vi "GetExecutableConfigurationFilePath.vi"(8 "Error In":errorcluster, 10 "Application Name":string, 11 "VI Path":path) -> (0 "Error Out":errorcluster, 3 "Executable Config File Path":path)   [LabVIEW 2012, in "LV-Utilities.lvlib"]
uses:
  LV-Utilities.lvlib
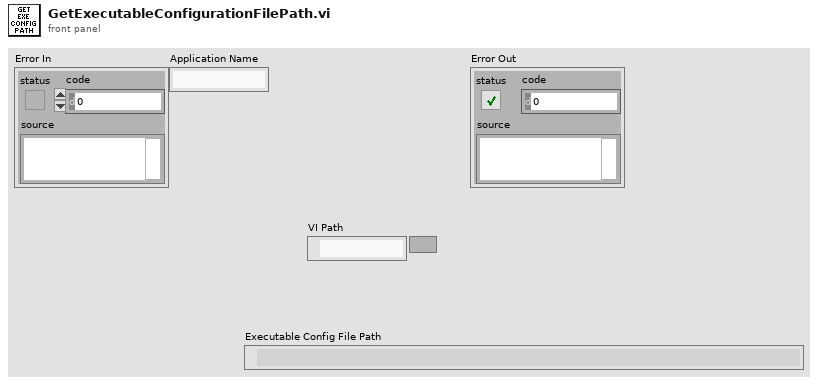
[diagram p1: front panel]
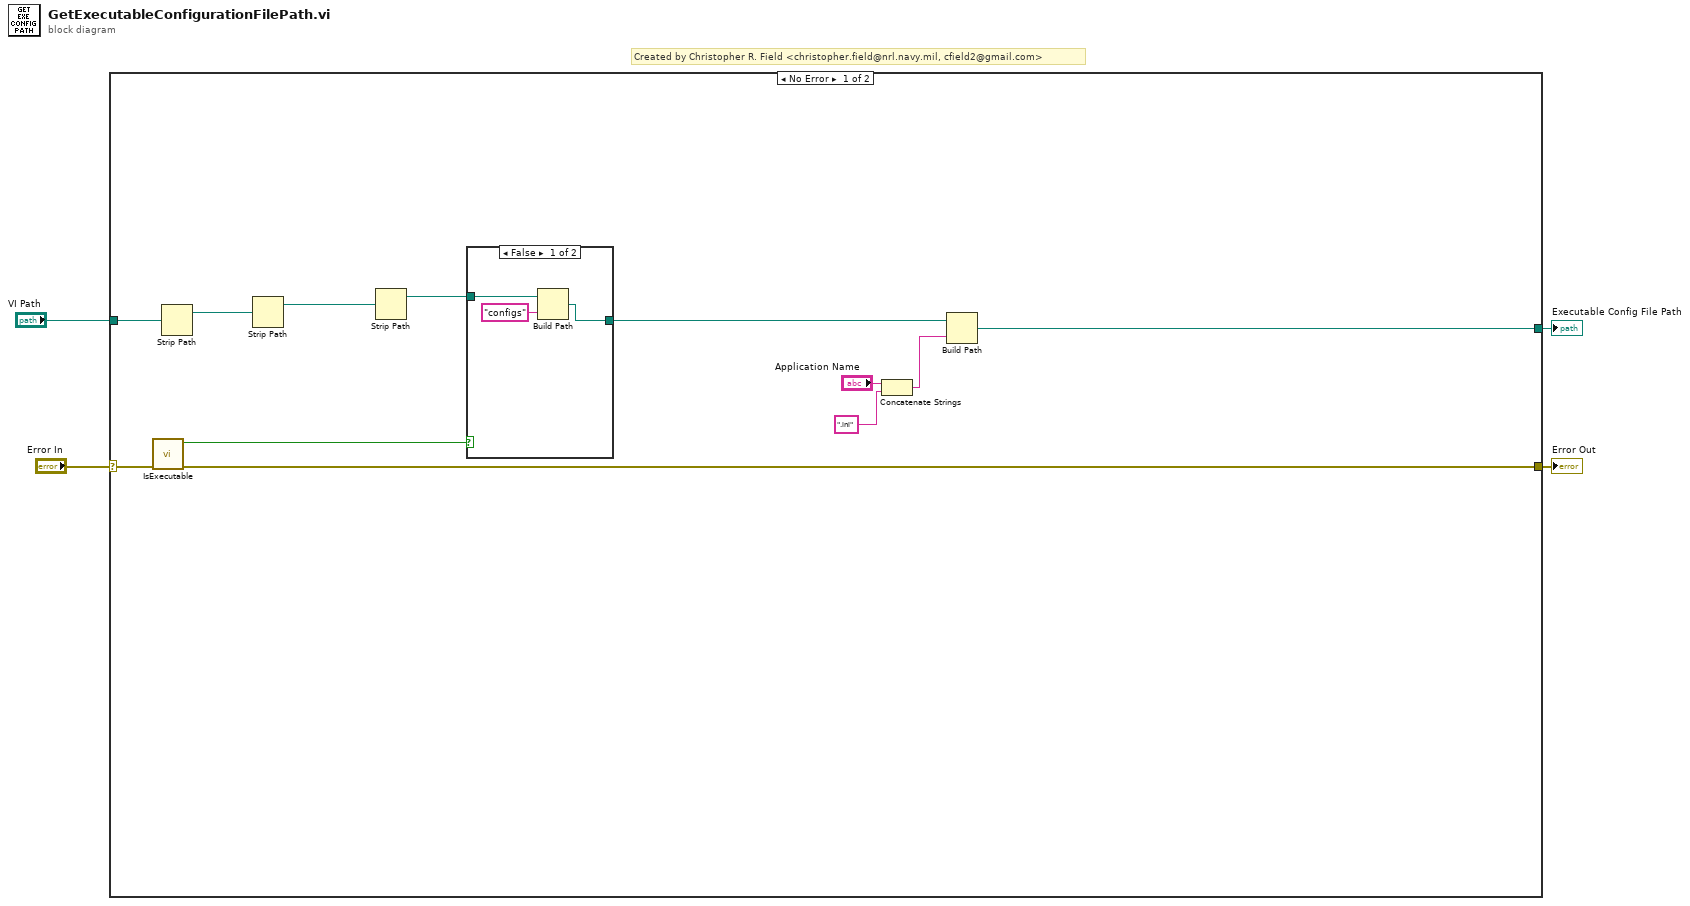
[diagram p0: block diagram]
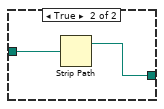
[diagram p2: hidden frame]
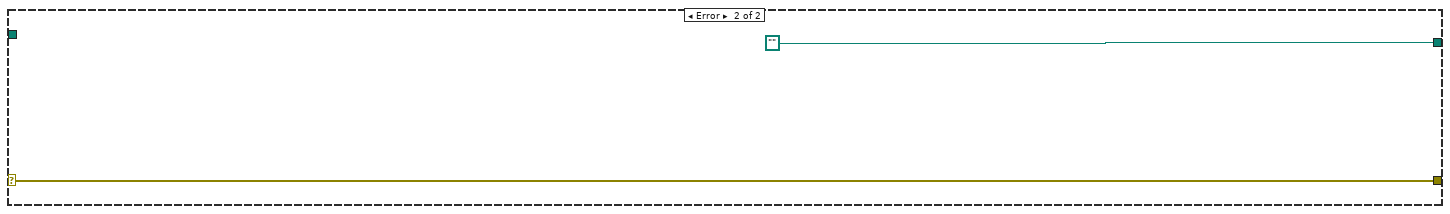
[diagram p3: hidden frame]
diagram:
  # "Created by Christopher R. Field <christopher.field@nrl.navy.mil, cfield2@gmail.com>"
  n1 = case shown="No Error" "Error In" {
    selector: "Error In" -> [w13 w22]
    tunnel: "VI Path" -> [w16 _]
    tunnel: [w11 w22] -> w2
    tunnel: [w10 path ""] -> w1
    frame No Error {
      n2 = call "IsExecutable.vi"("Error In"=w13) -> ("Error Out"=w11:errorcluster, "Executable?"=w15:bool)  [unwired: 9 in]
      n3 = Strip Path(path=w16) -> (stripped path=w6:path)  [unwired: 1 out]
      n4 = Strip Path(path=w6) -> (stripped path=w7:path)  [unwired: 1 out]
      n5 = Strip Path(path=w7) -> (stripped path=w5:path)  [unwired: 1 out]
      n6 = case shown="False" w15 {
        tunnel: [w18 w20] -> w14
        tunnel: w5 -> [w17 w21]
        frame False {
          n7 = Build Path(base path=w17, name or relative path="configs") -> (appended path=w18:path)
        }
        frame True {
          n8 = Strip Path(path=w21) -> (stripped path=w20:path)  [unwired: 1 out]
        }
      }
      n9 = Concatenate Strings("Application Name", ".ini" ("name or relative path")) -> (w9:string)
      n10 = Build Path(base path=w14, name or relative path=w9) -> (appended path=w10:path)
    }
    frame Error {
    }
  }
  "Error Out" <- w2
  "Executable Config File Path" <- w1
